vi "Call Matlab Function.vi"(7 "Timestamp":bool, 8 "error in (no error)":errorcluster, 9 "Matlab Param Array":cluster{"Name":string, "Data":variant}[](array[cluster]), 10 "Function name":string="netStartTrial", 11 "TrialBasedExperiment in":refnum<class "MatlabExperiment.lvclass">) -> (0 "error out":errorcluster, 1 "Return value struct":cluster{"Name":string, "Data":variant}[](array[cluster]), 2 "Return value I32":i32, 3 "TrialBasedExperiment out":refnum<class "MatlabExperiment.lvclass">)   [LabVIEW 2014, in "AcquisitionCoreObjects.lvlib" / "MatlabExperiment.lvclass"]
uses:
  MatlabExperiment.lvclass
  Matlab API/Matlab API.lvlib
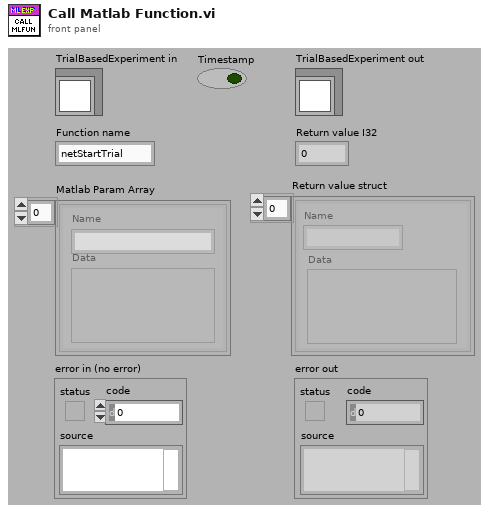
[diagram p1: front panel]
types:
  T1 = enum16{"Get Time", "Get Elapsed Time", "Reset Elapsed Time"}
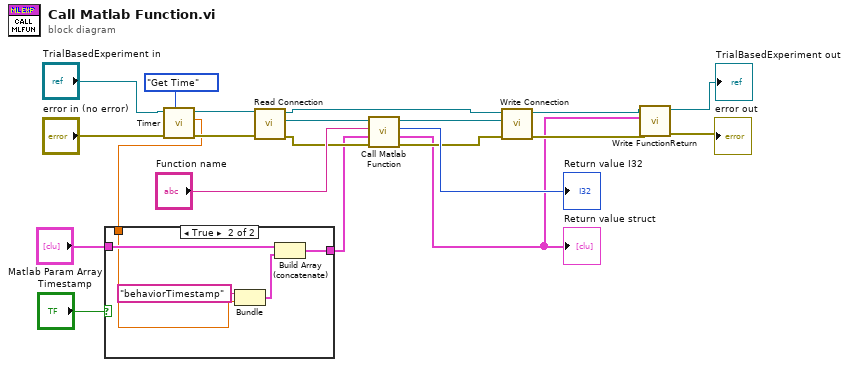
[diagram p0: block diagram]
diagram:
  n1 = call-dynamic "Timer.vi"("Method"=T1."Get Time", "error in (no error)"="error in (no error)", "BehaviorData in"="TrialBasedExperiment in") -> ("error out"=w4:errorcluster, "Time"=w1:dbl, "BehaviorData out"=w5:refnum<class "MatlabExperiment.lvclass">)  [unwired: 5 in, 1 out]
  n2 = case shown="True" "Timestamp" {
    tunnel: "Matlab Param Array" -> [w22 w25]
    tunnel: [w22 w24] -> w13
    tunnel: w1 -> [_ w23]
    frame False {
    }
    frame True {
      n3 = Bundle("behaviorTimestamp", "Time"=w23) -> (w26:cluster{string, "Time":dbl})  [unwired: 1 out]
      n4 = Build Array (concatenate)(w25, w26) -> (w24:cluster{"Name":string, "Data":variant}[])
    }
  }
  n5 = call-dynamic "Read Connection.vi"("error in (no error)"=w4, "TrialBasedExperiment in"=w5) -> ("error out"=w18:errorcluster, "Connection"=w20:refnum<k5>, "TrialBasedExperiment out"=w21:refnum<class "MatlabExperiment.lvclass">)  [unwired: 7 in]
  n6 = call "Call Matlab Function.vi"("error in (no error)"=w18, "Matlab Param Array"=w13, "Function name"="Function name", "TCP Network Connection Refnum"=w20) -> ("error out"=w15:errorcluster, "Return value struct"=w7:cluster{"Name":string, "Data":variant}[], "Return value I32"=→"Return value I32":i32, "connection ID out"=w16:refnum<k5>)  [unwired: 4 out]
  "Return value struct" <- w7
  n7 = call-dynamic "Write Connection.vi"("error in (no error)"=w15, "Connection"=w16, "TrialBasedExperiment in"=w21) -> ("error out"=w10:errorcluster, "TrialBasedExperiment out"=w11:refnum<class "MatlabExperiment.lvclass">)  [unwired: 7 in]
  n8 = call-dynamic "Write FunctionReturn.vi"("error in (no error)"=w10, "FunctionReturn"=w7, "MatlabExperiment in"=w11) -> ("error out"=→"error out":errorcluster, "MatlabExperiment out"=→"TrialBasedExperiment out":refnum<class "MatlabExperiment.lvclass">)  [unwired: 7 in]
